vi "Configure Number of Envelopes [MmW] Core.vi"(8 "error in (no error)":errorcluster, 10 "number of envelopes (8)":i32=8, 11 "IVI_Scope in":refnum<class "IVI_Scope.lvclass">) -> (0 "error out":errorcluster, 3 "IVI_Scope out":refnum<class "IVI_Scope.lvclass">)   [LabVIEW 2015, in "IVI_Scope.lvlib" / "IVI_Scope.lvclass"]
doc: "When you set the acquisition type to IVISCOPE_VAL_ENVELOPE, the oscilloscope acquires multiple waveforms. After each waveform acquisition, the oscilloscope keeps the minimum and maximum values it finds for each element in the waveform record. This VI configures the number of waveforms the oscilloscope acquires and analyzes to create the minimum and maximum waveforms. After the oscilloscope acquires as many waveforms as you specify, it returns to the idle state."
uses:
  IVI_Scope.lvclass
  IVI_Scope.lvclass/IVI_Scope.ctl
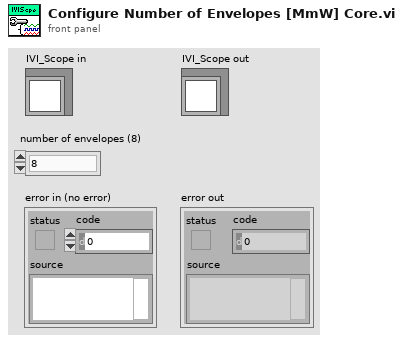
[diagram p1: front panel]
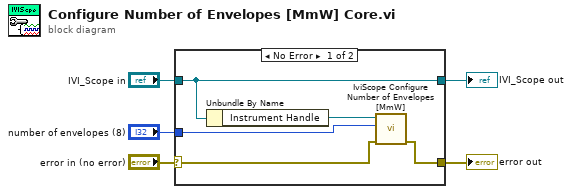
[diagram p0: block diagram]
diagram:
  n1 = case shown="No Error" "error in (no error)" {
    selector: "error in (no error)" -> [w8 w12]
    tunnel: [w7 w12] -> w4
    tunnel: [w10 w11] -> w2
    tunnel: "IVI_Scope in" -> [w10 w11]
    tunnel: "number of envelopes (8)" -> [w6 _]
    frame No Error {
      n2 = Unbundle By Name(w10) -> ("Instrument Handle"=w9:refnum<k15>)
      n3 = call <vilib>:"IviScope Configure Number of Envelopes [MmW].vi"("error in (no error)"=w8, "number of envelopes (8)"=w6, "instrument handle"=w9) -> ("error out"=w7:errorcluster)  [unwired: 7 in, 1 out]
    }
    frame Error {
    }
  }
  "error out" <- w4
  "IVI_Scope out" <- w2
